vi "Calibrate.vi"() -> ()   [LabVIEW 2011, in "Kinect_API.lvlib"]
uses:
  Kinect_API.lvlib
panel:
  out "output variable":dbl
  in  "input variable":u16[][](array[numeric])
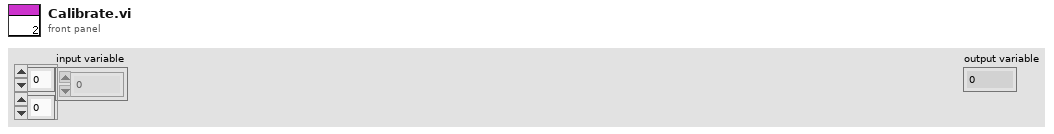
[diagram p1: front panel]
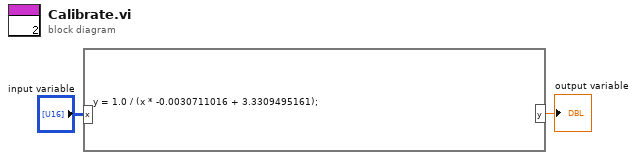
[diagram p0: block diagram]
diagram:
  n1 = formula code="y = 1.0 / (x * -0.0030711016 + 3.3309495161);"("x"="input variable") -> ("y"=→"output variable":dbl)
